vi "Generic command handler.vi"(8 "error in (no error)":errorcluster, 10 "Message in":refnum<class "GenericMessage.lvclass">, 11 "Waveform in":refnum<class "Waveform.lvclass">) -> (0 "error out":errorcluster, 2 "value":string, 3 "Waveform out":refnum<class "Waveform.lvclass">)   [LabVIEW 2012, in "Waveform.lvclass"]
doc: "The generic_command_handler processes the command 'generic'. Commands which are not part of the predefined list of commands fall under the 'generic' command for special activity."
uses:
  Waveform.lvclass
  <vilib>/Distrio/Murmex/GenericMessage/GenericMessage.lvclass
  <vilib>/Distrio/Murmex/Murmex/Murmex.lvclass
  Waveform.lvclass/Waveform.ctl
  <vilib>/Distrio/Murmex/Message/Add or replace parameter.vi
  <vilib>/DAQmx/configure/trigger.llb/DAQmx Start Trigger (None).vi
  <vilib>/Distrio/Murmex/Message/Message.lvclass
  <resource>/objmgr/daqmx.rc
panel:
  # "This method is called when the GENERIC\ntrigger is sent. \n\nOverride this method when your component needs to\nrespond to this trigger. \n\nCall parent for proper implementation"
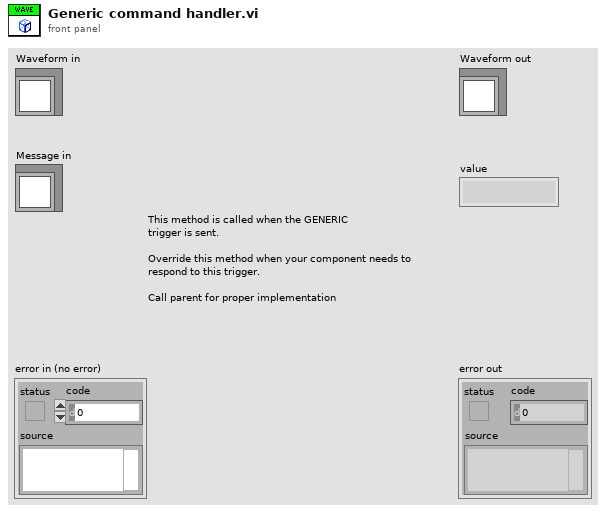
[diagram p1: front panel]
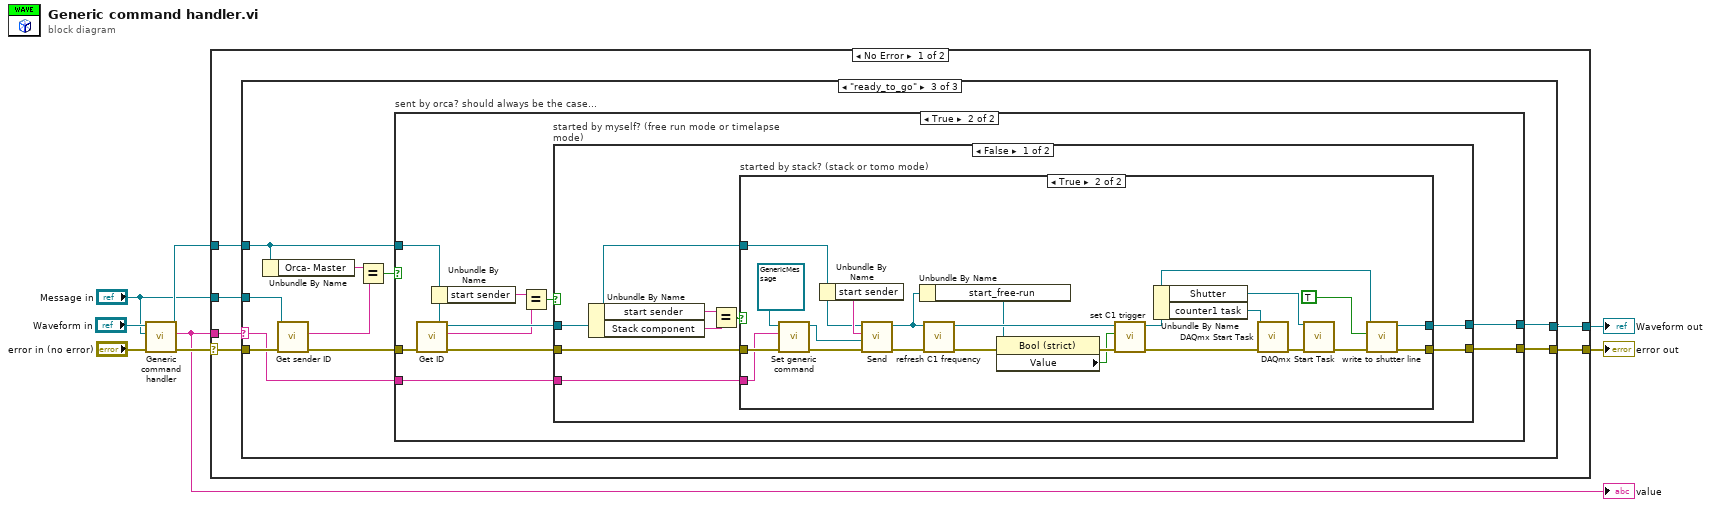
[diagram p0: block diagram]
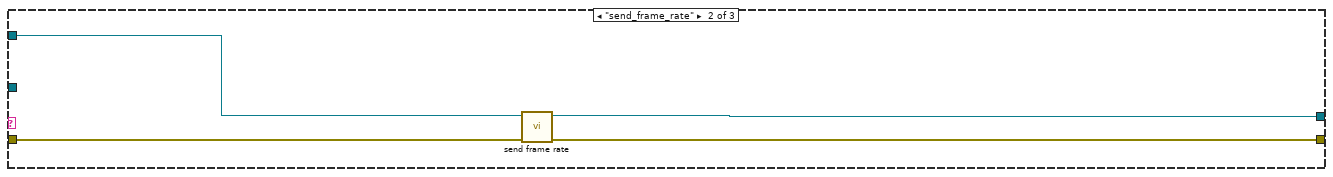
[diagram p3: hidden frame]
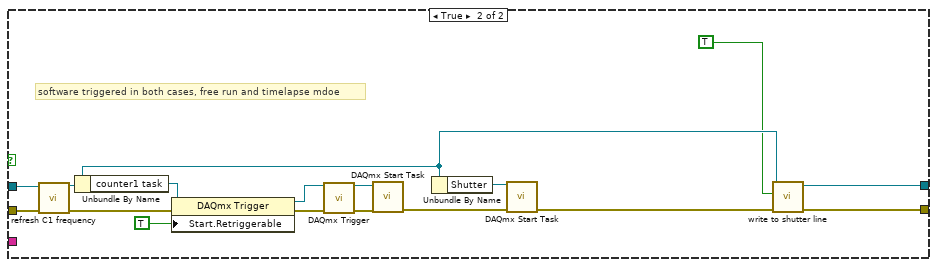
[diagram p6: hidden frame]
diagram:
  n1 = call-parent "Generic command handler.vi"("error in (no error)"="error in (no error)", "Message in"="Message in", "Murmex in"="Waveform in") -> ("error out"=w6:errorcluster, "value"=w2:string, "Murmex out"=w4:refnum<class "Waveform.lvclass">)  [unwired: 6 in]
  "value" <- w2
  n2 = case shown="No Error" w6 {
    selector: w6 -> [w14 w93]
    tunnel: [w11 w93] -> w5
    tunnel: w4 -> [w12 w92]
    tunnel: [w10 w92] -> w3
    tunnel: w2 -> [w13 _]
    tunnel: "Message in" -> [w9 _]
    frame No Error {
      n3 = case shown="\"ready_to_go\"" w13 {
        selector: w13 -> [_ _ w29]
        tunnel: w14 -> [w16 w20 w30]
        tunnel: w12 -> [w15 w19 w24]
        tunnel: [w16 w17 w28] -> w11
        tunnel: [w15 w18 w27] -> w10
        tunnel: w9 -> [_ _ w25]
        frame "False", Default {
        }
        frame "send_frame_rate" {
          n4 = call-dynamic "send frame rate.vi"("error in (no error)"=w20, "Waveform in"=w19) -> ("error out"=w17:errorcluster, "Waveform out"=w18:refnum<class "Waveform.lvclass">)  [unwired: 8 in]
        }
        frame "ready_to_go" {
          n5 = Unbundle By Name(w24) -> ("Orca- Master"=w23:string)
          n6 = call <vilib>:"Get sender ID.vi"("error in (no error)"=w30, "Message in"=w25) -> ("error out"=w26:errorcluster, "sender"=w21:string)  [unwired: 7 in, 1 out]
          n7 = Equal?(x=w23, y=w21) -> (x = y?=w22:bool)
          n8 = case "sent by orca? should always be the case..." shown="True" w22 {
            tunnel: w29 -> [_ w33]
            tunnel: [w32 w41] -> w28
            tunnel: [w31 w40] -> w27
            tunnel: w26 -> [w32 w42]
            tunnel: w24 -> [w31 w36]
            frame False {
            }
            frame True {
              n9 = call <vilib>:"Get ID.vi"("error in (no error)"=w42, "Murmex in"=w36) -> ("error out"=w37:errorcluster, "component id"=w34:string, "Murmex out"=w35:refnum<class "Waveform.lvclass">)  [unwired: 7 in]
              n10 = Unbundle By Name(w36) -> ("start sender"=w39:string)
              n11 = Equal?(x=w39, y=w34) -> (x = y?=w38:bool)
              n12 = case "started by myself? (free run mode or timelapse mode)" shown="False" w38 {
                tunnel: w37 -> [w47 w89]
                tunnel: [w46 w77] -> w41
                tunnel: [w45 w78] -> w40
                tunnel: w35 -> [w44 w87]
                tunnel: w33 -> [w43 _]
                frame False {
                  n13 = Unbundle By Name(w44) -> ("start sender"=w50:string, "Stack component"=w48:string)
                  n14 = Equal?(x=w50, y=w48) -> (x = y?=w49:bool)
                  n15 = case "started by stack? (stack or tomo mode)" shown="True" w49 {
                    tunnel: [w52 w59] -> w46
                    tunnel: [w51 w57] -> w45
                    tunnel: w47 -> [w52 w72]
                    tunnel: w44 -> [w51 w55]
                    tunnel: w43 -> [_ w71]
                    frame False {
                    }
                    frame True {
                      n16 = call <vilib>:"Set generic command.vi"("error in (no error)"=w72, "generic command"=w71, "GenericMessage in"=refnum<class "GenericMessage.lvclass"> refnum ("Distrio Murmex 1.2:GenericMessage")) -> ("error out"=w54:errorcluster, "GenericMessage out"=w73:refnum<class "GenericMessage.lvclass">)  [unwired: 7 in]
                      n17 = Unbundle By Name(w55) -> ("start sender"=w74:string)
                      n18 = call <vilib>:"Send.vi"("error in (no error)"=w54, "Message"=w73, "recipient"=w74, "Murmex in"=w55) -> ("error out"=w58:errorcluster, "Murmex out"=w56:refnum<class "Waveform.lvclass">)  [unwired: 6 in]
                      n19 = Unbundle By Name(w56) -> ("start_free-run"=w61:refnum<vi>)
                      n20 = call-dynamic "refresh C1 frequency.vi"("error in (no error)"=w58, "Waveform in"=w56) -> ("error out"=w63:errorcluster, "Waveform out"=w65:refnum<class "Waveform.lvclass">)  [unwired: 8 in]
                      n21 = property class="Bool (strict)"(reference=w61, error in=w63) -> (error out=w62:errorcluster, "Value"=w60:bool)  [unwired: 1 out]
                      n22 = call-dynamic "set C1 trigger.vi"("error in (no error)"=w62, "free run?"=w60, "Waveform in"=w65) -> ("error out"=w67:errorcluster, "Waveform out"=w64:refnum<class "Waveform.lvclass">)  [unwired: 7 in]
                      n23 = Unbundle By Name(w64) -> ("Shutter"=w70:refnum<k21>, "counter1 task"=w68:refnum<k21>)
                      n24 = call <vilib>:"DAQmx Start Task.vi"("task/channels in"=w68, "error in"=w67) -> ("error out"=w69:errorcluster)  [unwired: 12 in, 1 out]
                      n25 = call <vilib>:"DAQmx Start Task.vi"("task/channels in"=w70, "error in"=w69) -> ("error out"=w66:errorcluster)  [unwired: 12 in, 1 out]
                      n26 = call-dynamic "write to shutter line.vi"("error in (no error)"=w66, "data"=TRUE, "Waveform in"=w64) -> ("error out"=w59:errorcluster, "Waveform out"=w57:refnum<class "Waveform.lvclass">)  [unwired: 7 in]
                    }
                  }
                }
                frame True {
                  # "software triggered in both cases, free run and timelapse mdoe"
                  n27 = call-dynamic "refresh C1 frequency.vi"("error in (no error)"=w89, "Waveform in"=w87) -> ("error out"=w84:errorcluster, "Waveform out"=w80:refnum<class "Waveform.lvclass">)  [unwired: 8 in]
                  n28 = Unbundle By Name(w80) -> ("counter1 task"=w85:refnum<k21>)
                  n29 = property class="DAQmx Trigger"(reference=w85, error in=w84, "Start.Retriggerable"=TRUE) -> (reference out=w82:refnum<k21>, error out=w83:errorcluster)
                  n30 = call-poly <vilib>:"DAQmx Trigger.vi"("task/channels in"=w82, "error in"=w83) -> ("task out"=w79:refnum<k21>, "error out"=w81:errorcluster)  [unwired: 12 in]
                  n31 = call <vilib>:"DAQmx Start Task.vi"("task/channels in"=w79, "error in"=w81) -> ("error out"=w90:errorcluster)  [unwired: 12 in, 1 out]
                  n32 = Unbundle By Name(w80) -> ("Shutter"=w91:refnum<k21>)
                  n33 = call <vilib>:"DAQmx Start Task.vi"("task/channels in"=w91, "error in"=w90) -> ("error out"=w88:errorcluster)  [unwired: 12 in, 1 out]
                  n34 = call-dynamic "write to shutter line.vi"("error in (no error)"=w88, "data"=TRUE, "Waveform in"=w80) -> ("error out"=w77:errorcluster, "Waveform out"=w78:refnum<class "Waveform.lvclass">)  [unwired: 7 in]
                }
              }
            }
          }
        }
      }
    }
    frame Error {
    }
  }
  "error out" <- w5
  "Waveform out" <- w3
